vi "DE_Check Inputs.vi"(6 "DE settings":T3={"population size"=10, "scale factor"=0.9, "crossover probability"=0.95, "bound mapping method"=1, "mutation method"=0, "crossover method"=0} {"crossover method" items=["Uniform", "Exponential"]; "mutation method" items=["Random", "Either Or", "Best", "Target to Best"]; "bound mapping method" items=["None", "Random between Bounds and Values", "Re-Initialize"]}, 8 "error in (no error)":errorcluster, 9 "Beginning State":T1, 10 "Bounds":cluster{"Min":dbl[], "Max":dbl[]}, 11 "Init Parameters":dbl[][](array[numeric])) -> (0 "error out":errorcluster)   [LabVIEW 2020, in "NI_AAL_GlobalOptimization.lvlib"]
uses:
  <vilib>/gmath/NI_AAL_GlobalOptimization.lvlib
  <vilib>/gmath/GlobalOptimization.llb/DE_Settings.ctl
  <vilib>/gmath/GlobalOptimization.llb/DE_Bound Mapping Method.ctl
  <vilib>/gmath/GlobalOptimization.llb/DE_Mutation Method.ctl
  <vilib>/gmath/GlobalOptimization.llb/DE_Crossover Method.ctl
  <vilib>/gmath/GlobalOptimization.llb/DE_State.ctl
  <vilib>/gmath/GlobalOptimization.llb/DE_Population.ctl
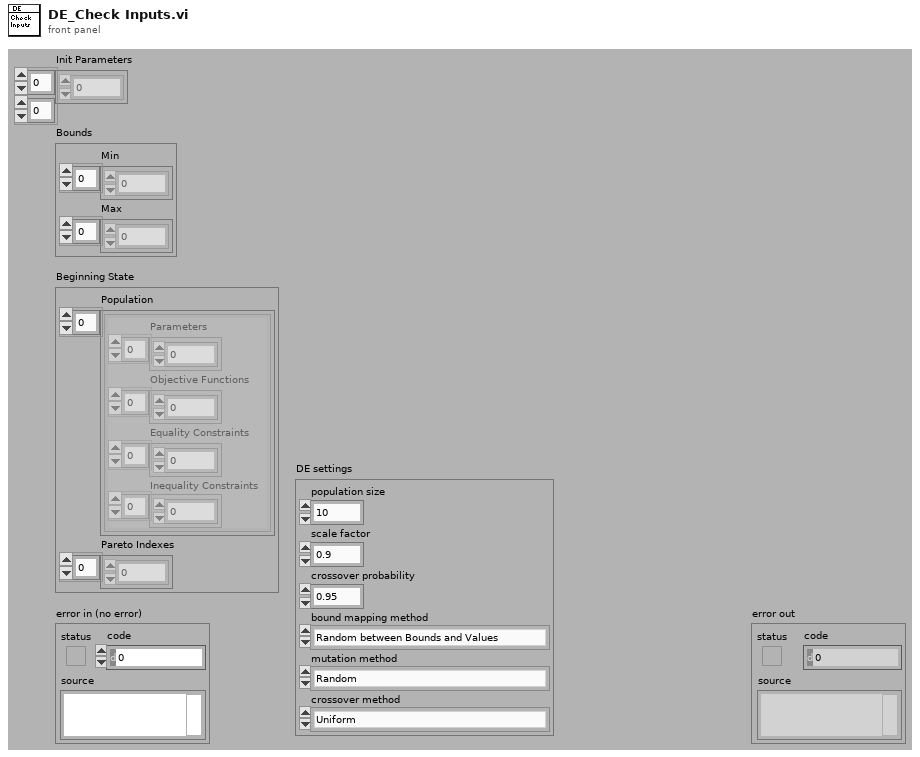
[diagram p1: front panel]
types:
  T1 = typedef "NI_AAL_GlobalOptimization.lvlib/DE_State.ctl" = cluster{"Population":T2[], "Pareto Indexes":i32[]}
  T2 = typedef "NI_AAL_GlobalOptimization.lvlib/DE_Population.ctl" = cluster{"Parameters":dbl[], "Objective Functions":dbl[], "Equality Constraints":dbl[], "Inequality Constraints":dbl[]}
  T3 = typedef "NI_AAL_GlobalOptimization.lvlib/DE_Settings.ctl" = cluster{"population size":i32, "scale factor":dbl, "crossover probability":dbl, "bound mapping method":T4, "mutation method":T5, "crossover method":T6}
  T4 = typedef "NI_AAL_GlobalOptimization.lvlib/DE_Bound Mapping Method.ctl" = u16
  T5 = typedef "NI_AAL_GlobalOptimization.lvlib/DE_Mutation Method.ctl" = u16
  T6 = typedef "NI_AAL_GlobalOptimization.lvlib/DE_Crossover Method.ctl" = u16
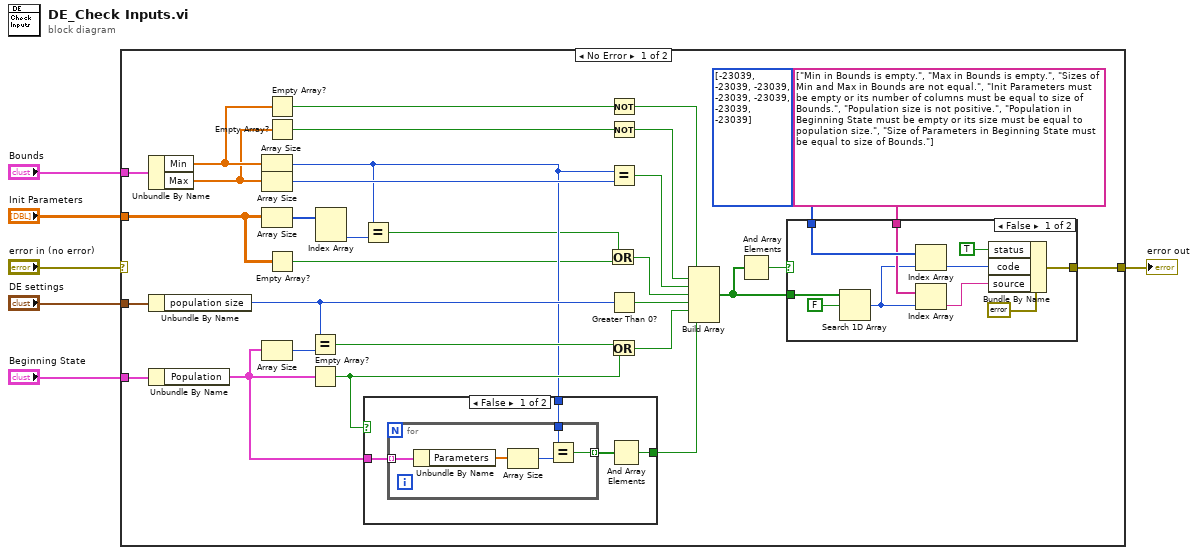
[diagram p0: block diagram]
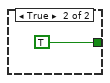
[diagram p3: hidden frame]
diagram:
  n1 = case shown="No Error" "error in (no error)" {
    selector: "error in (no error)" -> [_ w58]
    tunnel: "Init Parameters" -> [w21 _]
    tunnel: "DE settings" -> [w37 _]
    tunnel: "Bounds" -> [w36 _]
    tunnel: [w23 w58] -> w2
    tunnel: "Beginning State" -> [w34 _]
    frame No Error {
      n2 = Unbundle By Name(w36) -> ("Min"=w14:dbl[], "Max"=w10:dbl[])
      n3 = Unbundle By Name(w37) -> ("population size"=w31:i32)
      n4 = Unbundle By Name(w34) -> ("Population"=w29:T2[])
      n5 = Array Size(array=w14) -> (size(s)=w19:i32)
      n6 = Array Size(array=w10) -> (size(s)=w35:i32)
      n7 = Array Size(array=w21) -> (size(s)=w20:i32[])
      n8 = Array Size(array=w29) -> (size(s)=w33:i32)
      n9 = Empty Array?(array=w14) -> (empty?=w13:bool)
      n10 = Empty Array?(array=w10) -> (empty?=w11:bool)
      n11 = Empty Array?(array=w21) -> (empty?=w17:bool)
      n12 = Equal?(x=w31, y=w33) -> (x = y?=w32:bool)
      n13 = Empty Array?(array=w29) -> (empty?=w30:bool)
      n14 = Index Array(array=w20) -> (element #2=w15:i32)  [unwired: 2 in, 1 out]
      n15 = Equal?(x=w19, y=w15) -> (x = y?=w18:bool)
      n16 = case shown="False" w30 {
        tunnel: w29 -> [w51 _]
        tunnel: w19 -> [w50 _]
        tunnel: [w48 TRUE] -> w26
        frame False {
          n17 = for {
            tunnel: w51 -> [w56] mode=indexing
            tunnel: w50 -> [w53]
            tunnel: [w52] -> w49 mode=indexing
            n18 = Unbundle By Name(w56) -> ("Parameters"=w55:dbl[])
            n19 = Array Size(array=w55) -> (size(s)=w54:i32)
            n20 = Equal?(x=w53, y=w54) -> (x = y?=w52:bool)
          }
          n21 = And Array Elements(Boolean array=w49) -> (logical AND=w48:bool)
        }
        frame True {
        }
      }
      n22 = Or(x=w18, y=w17) -> (x .or. y?=w16:bool)
      n23 = Not(x=w13) -> (.not. x?=w12:bool)
      n24 = Not(x=w11) -> (.not. x?=w8:bool)
      n25 = Equal?(x=w19, y=w35) -> (x = y?=w9:bool)
      n26 = Greater Than 0?(x=w31) -> (x > 0?=w28:bool)
      n27 = Or(x=w32, y=w30) -> (x .or. y?=w27:bool)
      n28 = Build Array(w12, w8, w9, w16, w28, w27, w26) -> (w24:bool[])
      n29 = And Array Elements(Boolean array=w24) -> (logical AND=w25:bool)
      n30 = case shown="False" w25 {
        tunnel: w24 -> [w47 _]
        tunnel: [w44 _] -> w23
        tunnel: i32[] [-23039, -23039, -23039, -23039, -23039, -23039, -23039] -> [w41 _]
        tunnel: string[] ["Min in Bounds is empty.", "Max in Bounds is empty.", "Sizes of Min and Max in Bounds are not equal.", "Init Parameters must be empty or its number of columns must be equal to size of Bounds.", "Population size is not positive.", "Population in Beginning State must be empty or its size must be equal to population size.", "Size of Parameters in Beginning State must be equal to size of Bounds."] -> [w40 _]
        frame False {
          n31 = Search 1D Array(1D array=w47, element=FALSE) -> (index of element=w39:i32)  [unwired: 1 in]
          n32 = Index Array(array=w41, index=w39) -> (element=w42:i32)
          n33 = Index Array(array=w40, index=w39) -> (element=w38:string)
          n34 = Bundle By Name(cluster=errorcluster {"status"=FALSE, "code"=0, "source"=""} ("error IO"), "status"=TRUE, "code"=w42, "source"=w38) -> (w44:errorcluster)
        }
        frame True {
        }
      }
    }
    frame Error {
    }
  }
  "error out" <- w2
